vi "Set Dev Auto.vi"(8 "error in (no error)":errorcluster, 9 "firmware revision":string(combo), 10 "dev point auto (F/F)":T2, 11 "VISA resource name":refnum<visa-resource-name>) -> (0 "error out":errorcluster, 2 "bridge error":T1, 3 "VISA resource name out":refnum<visa-resource-name>)   [LabVIEW 2021, in "Andeen-Hagerling 2700A.lvlib"]
doc: "Set the deviation mode auto parameter.\n\nDuring each initialization of the deviation mode the DUT is\nmeasured resulting in a set of capacitance and loss values\nknown as the Initial Deviation Reading. These values may be\nused to automatically establish new Deviation Setpoint values.\nAlternatively, the Deviation Setpoints remain fixed at\ntheir previous values and the Initial Deviation Readings are\nused simply to verify that the DUT is within the previously\nspecified upper and lower boundaries."
uses:
  Andeen-Hagerling 2700A.lvlib
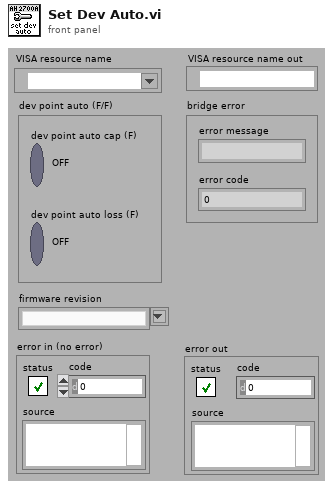
[diagram p1: front panel]
types:
  T1 = cluster{"error message":string, "error code":i32}
  T2 = cluster{"dev point auto cap (F)":bool, "dev point auto loss (F)":bool}
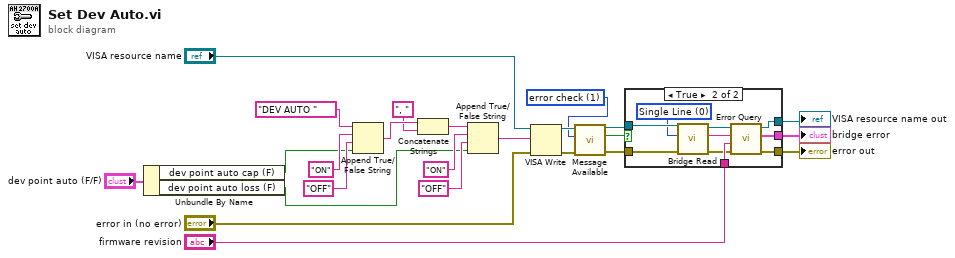
[diagram p0: block diagram]
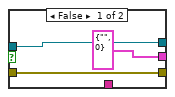
[diagram p2: hidden frame]
diagram:
  w1 = u16 1 items=["none", "error check", "multiline read", "infinite"] ("delay")
  n1 = Unbundle By Name("dev point auto (F/F)") -> ("dev point auto cap (F)"=w4:bool, "dev point auto loss (F)"=w3:bool)
  n2 = Append True/False String(1:w4, 2:"OFF" ("false string"), 3:"ON" ("true string"), 4:"DEV AUTO " ("command")) -> (0:w21:string)
  n3 = Concatenate Strings(w21, ", " ("command")) -> (w15:string)
  n4 = Append True/False String(1:w3, 2:"OFF" ("false string"), 3:"ON" ("true string"), 4:w15) -> (0:w16:string)
  n5 = VISA Write(VISA resource name="VISA resource name", write buffer=w16, error in (no error)="error in (no error)") -> (VISA resource name out=w11:refnum<visa-resource-name>, error out=w10:errorcluster)  [unwired: 1 out]
  n6 = call "Message Available.vi"("error in (no error)"=w10, "delay"=w1, "VISA resource name"=w11) -> ("error out"=w13:errorcluster, "message available"=w6:bool, "VISA resource name out"=w9:refnum<visa-resource-name>)  [unwired: 6 in]
  n7 = case shown="True" w6 {
    tunnel: w9 -> [w26 w32]
    tunnel: w13 -> [w27 w33]
    tunnel: "firmware revision" -> [_ w37]
    tunnel: [w27 w36] -> w8
    tunnel: [w26 w35] -> w7
    tunnel: [T1 {"error message"="", "error code"=0} ("bridge error") w34] -> w2
    frame False {
    }
    frame True {
      w28 = u16 0 items=["Single Line", "Multi-Line"] ("Multiline")
      n8 = call "Bridge Read.vi"("error in (no error)"=w33, "multiline"=w28, "VISA resource name"=w32) -> ("error out"=w29:errorcluster, "read buffer"=w30:string, "VISA resource name out"=w31:refnum<visa-resource-name>)  [unwired: 6 in]
      n9 = call "Error Query.vi"("error in (no error)"=w29, "firmware revision"=w37, "measurement line"=w30, "VISA resource name"=w31) -> ("error out"=w36:errorcluster, "bridge error"=w34:T1, "VISA resource name out"=w35:refnum<visa-resource-name>)  [unwired: 5 in]
    }
  }
  "VISA resource name out" <- w7
  "error out" <- w8
  "bridge error" <- w2
